vi "diagonalLength.vi"(8 "error in (no error)":errorcluster, 11 "Field in":refnum<class "Field.lvclass">) -> (0 "error out":errorcluster, 2 "diagonalLength":dbl, 3 "Field out":refnum<class "Field.lvclass">)   [LabVIEW 2020, in "Field.lvclass"]
uses:
  Field.lvclass
  Utilities_class/Utilities.lvclass
  Field.lvclass/Field.ctl
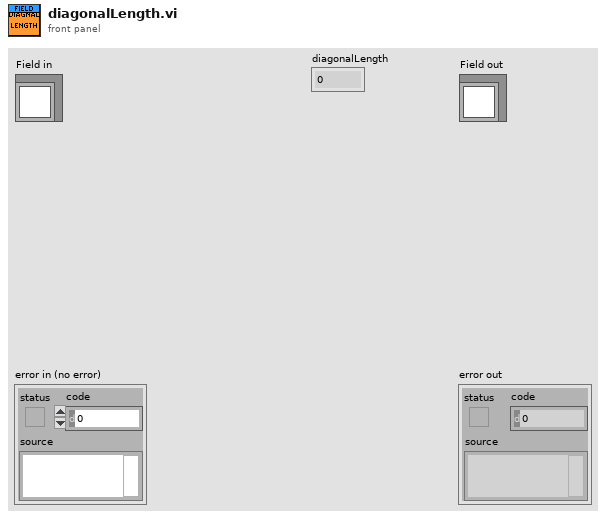
[diagram p1: front panel]
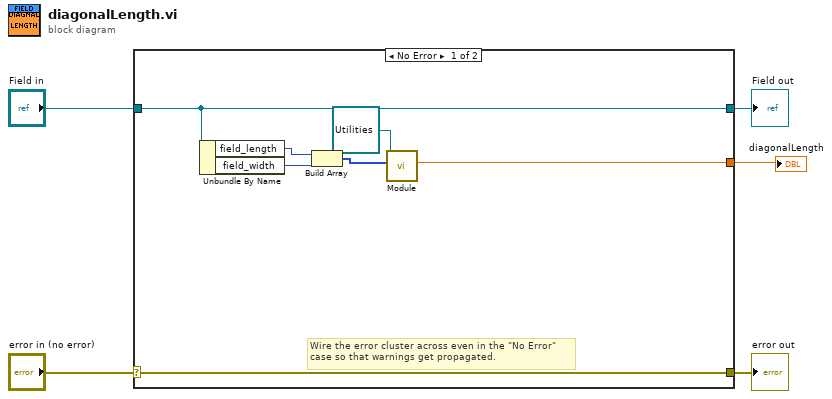
[diagram p0: block diagram]
diagram:
  n1 = case shown="No Error" "error in (no error)" {
    selector: "error in (no error)" -> [w12 w14]
    tunnel: [w12 w14] -> w4
    tunnel: [w11 w13] -> w2
    tunnel: "Field in" -> [w11 w13]
    tunnel: [w6 _] -> w1
    frame No Error {
      # "Wire the error cluster across even in the \"No Error\"\ncase so that warnings get propagated."
      n2 = Unbundle By Name(w11) -> ("field_length"=w10:i32, "field_width"=w9:i32)
      n3 = Build Array(w10, w9) -> (w8:i32[])
      n4 = call-dynamic "Module.vi"("2D vector"=w8, "Utilities in"=refnum<class "Utilities.lvclass"> refnum) -> ("Modulo"=w6:dbl)  [unwired: 7 in, 2 out]
    }
    frame Error {
    }
  }
  "error out" <- w4
  "Field out" <- w2
  "diagonalLength" <- w1
